vi "Ih_Image_FlipV.vi"(11 "2D array in":u32[][](array[numeric])) -> (3 "Flip V 2D array out":u32[][](array[numeric]))   [LabVIEW 2016]
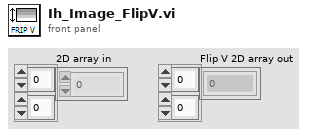
[diagram p1: front panel]
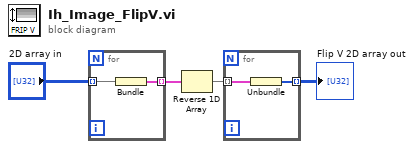
[diagram p0: block diagram]
diagram:
  n1 = for {
    tunnel: "2D array in" -> [w5] mode=indexing
    tunnel: [w6] -> w1 mode=indexing
    n2 = Bundle("2D array in"=w5) -> (w6:cluster{"2D array in":u32[]})  [unwired: 1 in]
  }
  n3 = Reverse 1D Array(array=w1) -> (reversed array=w2:cluster{"2D array in":u32[]}[])
  n4 = for {
    tunnel: w2 -> [w8] mode=indexing
    tunnel: [w7] -> w3 mode=indexing
    n5 = Unbundle(w8) -> ("2D array in"=w7:u32[])
  }
  "Flip V 2D array out" <- w3
